vi "ComputeUUSSize.vi"(3 "B Array Position":i32, 4 "BArray":i8[](array[numeric]), 5 "A Array Position":i32, 6 "A Array Num":i8[](array[numeric])) -> (0 "B Index":i32, 1 "A Index":i32, 2 "Loop Count":i32)   [LabVIEW 2025]
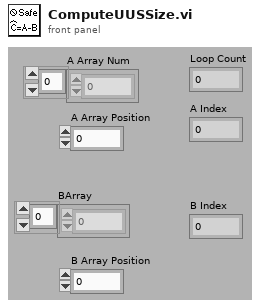
[diagram p1: front panel]
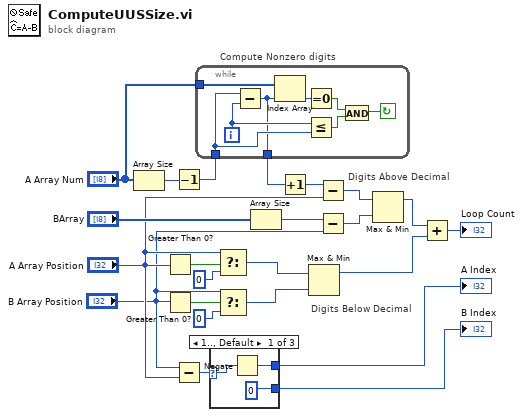
[diagram p0: block diagram]
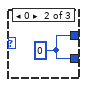
[diagram p2: hidden frame]
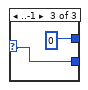
[diagram p3: hidden frame]
diagram:
  # "Digits Below Decimal"
  # "Digits Above Decimal"
  # "Compute Nonzero digits"
  n1 = Array Size(array="A Array Num") -> (size(s)=w17:i32)
  n2 = Greater Than 0?(x="A Array Position") -> (x > 0?=w22:bool)
  n3 = Greater Than 0?(x="B Array Position") -> (x > 0?=w21:bool)
  n4 = Decrement(x=w17) -> (x-1=w16:i32)
  n5 = Subtract(x="B Array Position", y="A Array Position") -> (x-y=w12:i32)
  n6 = while {
    tunnel: "A Array Num" -> [w26]
    tunnel: w16 -> [w28]
    tunnel: [w24] -> w15
    i -> [w31]
    stop <- w30 continue-if-true
    n7 = Subtract(x=w28, y=w31) -> (x-y=w24:i32)
    n8 = Index Array(array=w26, index=w24) -> (element=w25:i8)
    n9 = Equal To 0?(x=w25) -> (x = 0?=w29:bool)
    n10 = Less Or Equal?(x=w31, y=w28) -> (x <= y?=w27:bool)
    n11 = And(x=w29, y=w27) -> (x .and. y?=w30:bool)
  }
  n12 = case shown="1.., Default" w12 {
    selector: w12 -> [w32 _ w36]
    tunnel: [w33 w35 0] -> w10
    tunnel: [0 w35 w36] -> w11
    frame 1.., Default {
      n13 = Negate(x=w32) -> (-x=w33:i32)
    }
    frame 0 {
      w35 = 0
    }
    frame ..-1 {
    }
  }
  "A Index" <- w10
  "B Index" <- w11
  n14 = Select(t="A Array Position", s=w22, f=0) -> (s? t:f=w1:i32)
  n15 = Select(t="B Array Position", s=w21, f=0) -> (s? t:f=w2:i32)
  n16 = Array Size(array="BArray") -> (size(s)=w19:i32)
  n17 = Increment(x=w15) -> (x+1=w14:i32)
  n18 = Max & Min(x=w1, y=w2) -> (max(x,y)=w7:i32)  [unwired: 1 out]
  n19 = Subtract(x=w14, y="A Array Position") -> (x-y=w20:i32)
  n20 = Subtract(x=w19, y="B Array Position") -> (x-y=w13:i32)
  n21 = Max & Min(x=w20, y=w13) -> (max(x,y)=w6:i32)  [unwired: 1 out]
  n22 = Add(x=w6, y=w7) -> (x+y=→"Loop Count":i32)
